vi "Destroy.vi"(11 "Dev Panel in":refnum<class "Dev Panel.lvclass">) -> ()   [LabVIEW 2021, in "Dev Panel.lvclass"]
uses:
  Dev Panel.lvclass
  Dev Panel.lvclass/Dev Panel.ctl
  Actor/Event Actor/Event Actor.lvclass
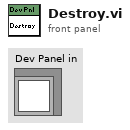
[diagram p1: front panel]
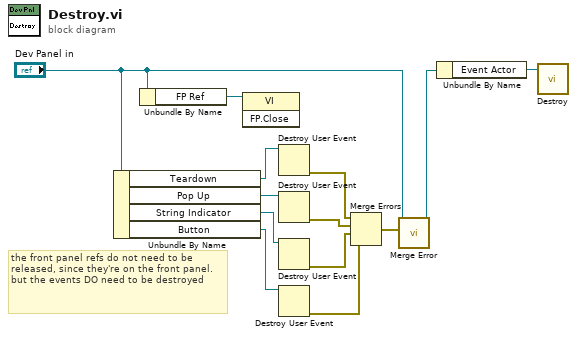
[diagram p0: block diagram]
diagram:
  # "the front panel refs do not need to be released, since they're on the front panel. but the events DO need to be destroyed"
  n1 = Unbundle By Name("Dev Panel in") -> ("Teardown"=w13:refnum<user-event>, "Pop Up"=w12:refnum<user-event>, "String Indicator"=w11:refnum<user-event>, "Button"=w10:refnum<user-event>)
  n2 = Unbundle By Name("Dev Panel in") -> ("FP Ref"=w9:refnum<vi>)
  n3 = invoke class="VI" method="FP.Close"(reference=w9) -> ()  [unwired: 2 in, 3 out]
  n4 = Destroy User Event(user event=w13) -> (error out=w8:errorcluster)  [unwired: 1 in]
  n5 = Destroy User Event(user event=w12) -> (error out=w7:errorcluster)  [unwired: 1 in]
  n6 = Destroy User Event(user event=w11) -> (error out=w6:errorcluster)  [unwired: 1 in]
  n7 = Destroy User Event(user event=w10) -> (error out=w5:errorcluster)  [unwired: 1 in]
  n8 = Merge Errors(w8, w7, w6, w5) -> (w1:errorcluster)
  n9 = call-dynamic "Merge Error.vi"("Error"=w1, "Set Error in"="Dev Panel in") -> ("Set Error out"=w2:refnum<class "Dev Panel.lvclass">)  [unwired: 9 in]
  n10 = Unbundle By Name(w2) -> ("Event Actor"=w4:refnum<class "Event Actor.lvclass">)
  n11 = call-dynamic "Destroy.vi"("Actor in"=w4) -> ()  [unwired: 11 in]
